vi "DIAG_STM Read Message.vi"   [LabVIEW 2013, in "Diagnostics Addon Engine.lvlib"]
doc: "This VI reads an incoming package of data from a host. This VI parses the package and extracts the data name and type as described in the meta data.\n\nFor the package to be parsed correctly, the meta data must be consistent in both the sender and the receiver. The data is packaged based on the existing meta data on the sender. \n\nUse the \"STM Read Meta Data\" and \"STM Write Meta Data\" VIs to ensure that both client and server have the same meta data.\n\nThe data is returned as a string. It is the responsibility of the user to cast it to the appropriate type."
uses:
  Diagnostics Addon Engine.lvlib
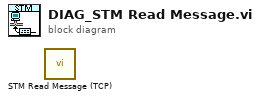
[diagram p0: block diagram]
diagram:
  n1 = call "STM Read Message (TCP).vi"() -> ()  [unwired: 6 in, 6 out]
